vi "EOL CAN_Get_Motor_Position.vi"(11 "NetworkObjHandle":T1) -> (1 "Position":u8 format="%02x", 2 "TxRx Data":string[][](array[string]), 3 "Response Good?":bool)   [LabVIEW 2018]
uses:
  <vilib>/nican/nican.llb/xobjhandle.ctl
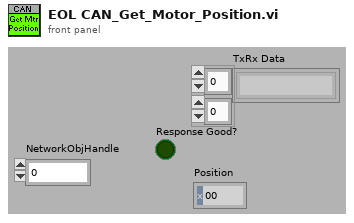
[diagram p1: front panel]
types:
  T1 = typedef "xobjhandle.ctl" = u32
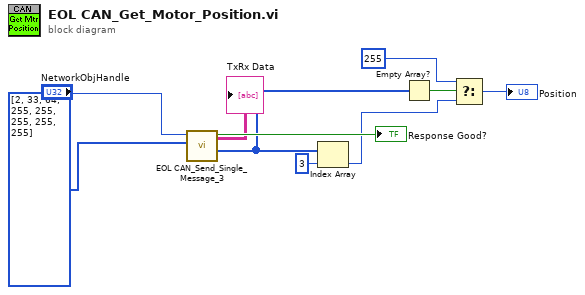
[diagram p0: block diagram]
diagram:
  n1 = call <userlib>:"EOL CAN_Send_Single_Message_3.vi"("Tx Msg"=u8[] [2, 33, 64, 255, 255, 255, 255, 255] ("Transmit Data"), "NetworkObjHandle"="NetworkObjHandle") -> ("Rx Message"=w6:u8[], "Response Good?"=→"Response Good?":bool, "TxRx Data"=→"TxRx Data":string[][])  [unwired: 6 in, 1 out]
  n2 = Index Array(array=w6, index=3) -> (element=w3:u8)
  n3 = Empty Array?(array=w6) -> (empty?=w5:bool)
  n4 = Select(t=u8 255 ("CAN Data"), s=w5, f=w3) -> (s? t:f=→"Position":u8)
